vi "GetSupportedVirtualChannel.vi"(11 "key values":T1[](array[typedef])) -> (2 "not supported virtual channels":string[](array[string]), 3 "supported virtual channels":string[](array[string]))   [LabVIEW 2017, in "McsaVirtualChannel.lvlib"]
uses:
  <vilib>/addons/InsightCM/Devices/Shared/Mcsa/McsaVirtualChannel/McsaVirtualChannel.lvlib
  <vilib>/addons/InsightCM/MessageBus/Base/controls/SectionKeyValues.ctl
  <vilib>/addons/InsightCM/MessageBus/Base/controls/KeyValuePair.ctl
  <vilib>/addons/InsightCM/Utilities/PropertyHelpers/PropertyHelpers.lvlib
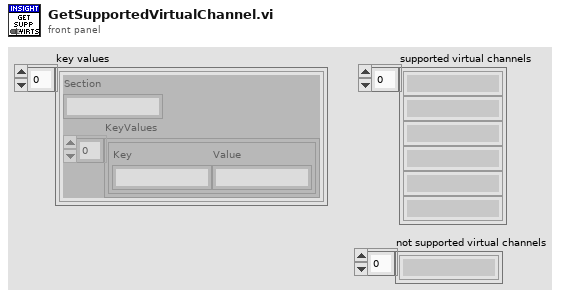
[diagram p1: front panel]
types:
  T1 = typedef "SectionKeyValues.ctl" = cluster{"Section":string, "KeyValues":T2[]}
  T2 = typedef "KeyValuePair.ctl" = cluster{"Key":string, "Value":string}
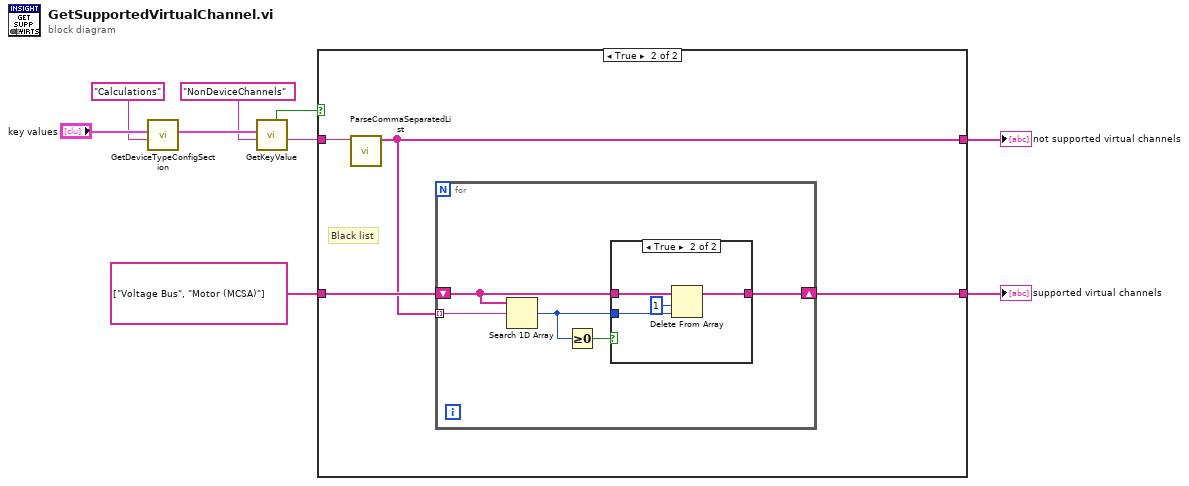
[diagram p0: block diagram]
diagram:
  n1 = call <vilib>:"GetDeviceTypeConfigSection.vi"("key"="Calculations", "key values"="key values") -> ("key value pairs out"=w7:T2[])  [unwired: 8 in, 1 out]
  n2 = call <vilib>:"GetKeyValue.vi"("key"="NonDeviceChannels", "key value pairs"=w7) -> ("value"=w4:string, "found"=w3:bool)  [unwired: 7 in, 1 out]
  n3 = case shown="True" w3 {
    tunnel: [w10 w12] -> w5
    tunnel: w4 -> [_ w14]
    tunnel: string[] ["Voltage Bus", "Motor (MCSA)"] ("Array") -> [w10 w13]
    tunnel: [_ w11] -> w2
    frame False {
    }
    frame True {
      # "Black list"
      n4 = call <vilib>:"ParseCommaSeparatedList.vi"("List"=w14) -> ("Array"=w11:string[])  [unwired: 10 in]
      n5 = for {
        tunnel: w11 -> [w19] mode=indexing
        shift-right: [w17] -> w12
        shift-left: w13 -> [w18]
        n6 = Search 1D Array(1D array=w18, element=w19) -> (index of element=w15:i32)  [unwired: 1 in]
        n7 = Greater Or Equal To 0?(x=w15) -> (x >= 0?=w16:bool)
        n8 = case shown="True" w16 {
          tunnel: w18 -> [w20 w23]
          tunnel: [w20 w22] -> w17
          tunnel: w15 -> [_ w21]
          frame False {
          }
          frame True {
            n9 = Delete From Array(array=w23, length=1, index=w21) -> (array with subset deleted=w22:string[])  [unwired: 1 out]
          }
        }
      }
    }
  }
  "supported virtual channels" <- w5
  "not supported virtual channels" <- w2
